vi "configuration UI.vi"() -> ()   [LabVIEW 2013, in "Tag Bus Web Interface editor node.lvclass"]
uses:
  Tag Bus Web Interface editor node.lvclass
  <vilib>/CEF_TreeControl/Node/NodeRef.ctl
  <vilib>/CEF_TreeControl/Node/NISE_CEF_Node.lvclass
  <vilib>/NI/AMC/Message Queue.ctl
  <vilib>/NI/AMC/Message.ctl
  <vilib>/NI/Tools/Keyed Array/KeyedArray.ctl
  <vilib>/CEF_TreeControl/Node/UserEventRef.ctl
  <vilib>/CEF_TreeControl/Controls/EventCluster.ctl
  <vilib>/NI/TBM Modules/TBWI/configuration/Tag Bus Web Interface configuration.lvclass
  <vilib>/NI/Module Execution Interface/Engine Configuration/engine configuration.lvclass
  <vilib>/NI/Tag Bus Data Framework/Configuration Editor/Classes/Engine Parent/Engine Parent Editor Node.lvclass
  <vilib>/NI/Tag Bus/tag/tag descriptor.lvclass
  <vilib>/NI/Tag Bus/tag/Data Type.ctl
  <vilib>/NI/Tag Bus/tag/tag descriptor.lvclass/tag descriptor.ctl
  <vilib>/NI/Tag Bus Module Framework/root configuration/TBM configuration.lvclass/TBM configuration.ctl
  <vilib>/NI/Tag Bus Module Framework/channel/channel classification.ctl
  <vilib>/NI/Tag Bus/tag/write tag name.vi
  <vilib>/NI/Tag Bus/tag/write data type.vi
  <vilib>/NI/Tag Bus Module Framework/root configuration/Read instance name.vi
  <vilib>/NI/Tag Bus/tag/read tag name.vi
  <vilib>/NI/Tag Bus Data Framework/Configuration Editor/Classes/Engine Parent/read engine configuration.vi
  <vilib>/NI/Tag Bus Data Framework/Configuration Editor/Classes/Module editor node/Read Module Configuration.vi
  <vilib>/NI/Tag Bus Module Framework/root configuration/create GUID.vi
  <vilib>/NI/Tag Bus Module Framework/root configuration/TBM configuration.lvclass
  <vilib>/NI/Tag Bus Module Framework/module configuration/TBM module configuration.lvclass
  <vilib>/NI/Tag Bus Data Framework/Configuration Editor/Classes/Module editor node/module editor node.lvclass
  <vilib>/CEF_TreeControl/NISE_CEF_TreeControl.lvlib
  <vilib>/NI/Tag Bus Module Framework/channel/TBM channel.lvclass
  <vilib>/NI/Tools/Keyed Array/Tools_KeyedArray.lvlib
  <vilib>/NI/AMC/AMC.lvlib
panel:
  in  "Tab Control":enum32{"Web Configuration"}(tab)
  in  "remove to":bool
  in  "add to":bool
  in  "remove from":bool
  in  "add from":bool
  in  "toTBWlist":i32(listbox)
  in  "fromTBWlist":i32(listbox)
  in  "avail tags":i32(listbox)=-1
  in  "Direction":enum32{"From TBWI", "To TBWI"}(radio)
  in  "user event":T1
  in  "main queue":T2
  in  "node ref":T3
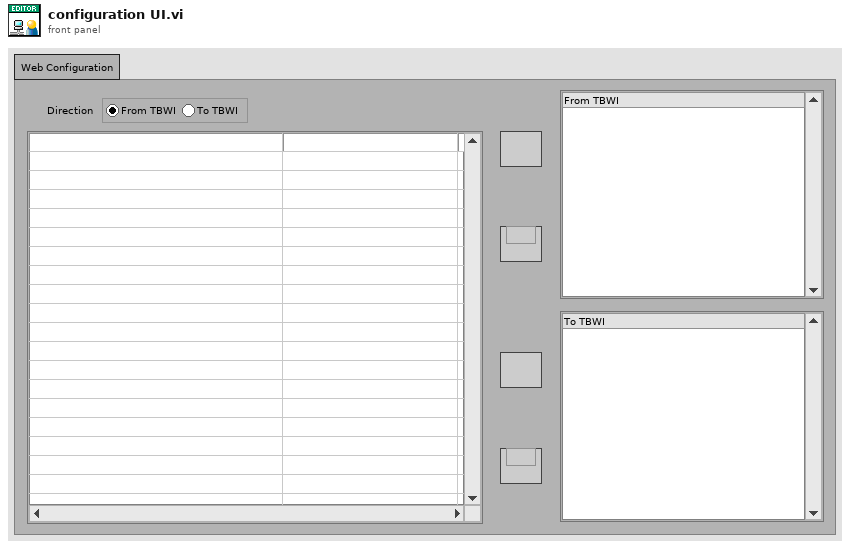
[diagram p1: front panel]
types:
  T1 = typedef "NISE_CEF_Node.lvclass/UserEventRef.ctl" = refnum<user-event>
  T2 = typedef "AMC.lvlib/Message Queue.ctl" = refnum<queue>
  T3 = typedef "NISE_CEF_Node.lvclass/NodeRef.ctl" = refnum<data-value>
  T4 = typedef "tag bus.lvlib/tag descriptor.lvclass/Data Type.ctl" = enum16{"Double", "Single", "I64", "I32", "I16", "I8", "U64", "U32", "U16", "U8", "Boolean", "String", "Array of Double", "Array of Single", "Array of I64", "Array of I32", "Array of I16", "Array of I8", "Array of U64", "Array of U32", "Array of U16", "Array of U8", "Array of Boolean", "Array of String"}
  T5 = typedef "NISE_CEF_TreeControl.lvlib/EventCluster.ctl" = cluster{"command":string, "data":string}
  T6 = enum8{"Enabled", "Disabled", "Disabled and Grayed Out"}
  T7 = typedef "TBM channel.lvclass/channel classification.ctl" = enum16{"input data", "output data", "processing parameter", "processing result"}
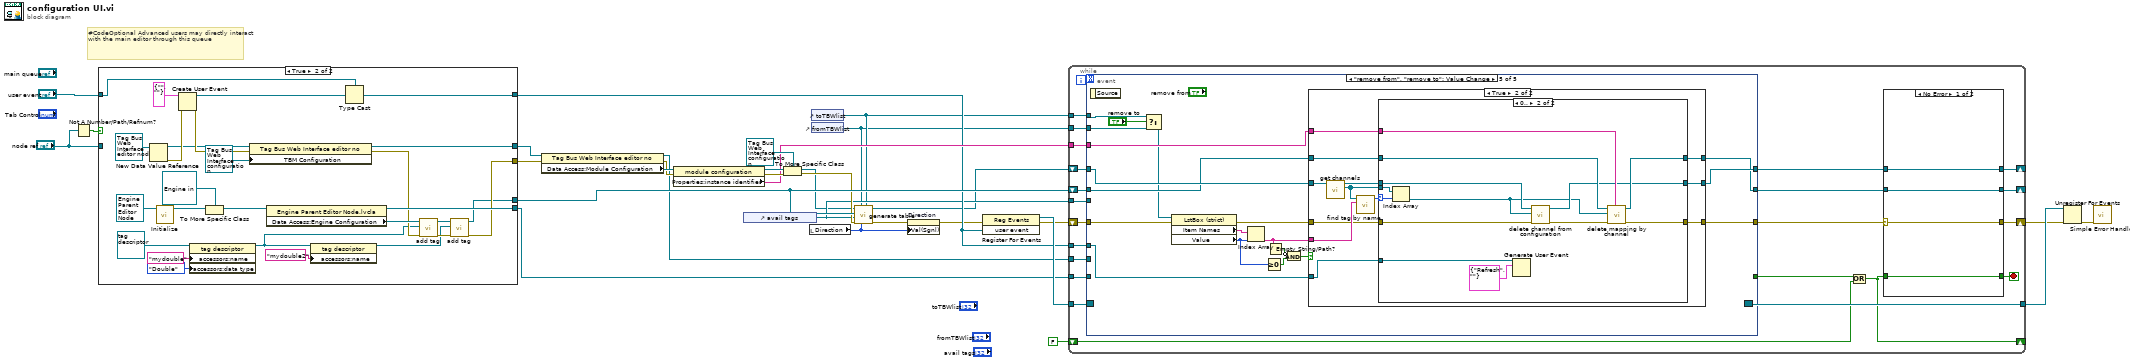
[diagram p0: block diagram]
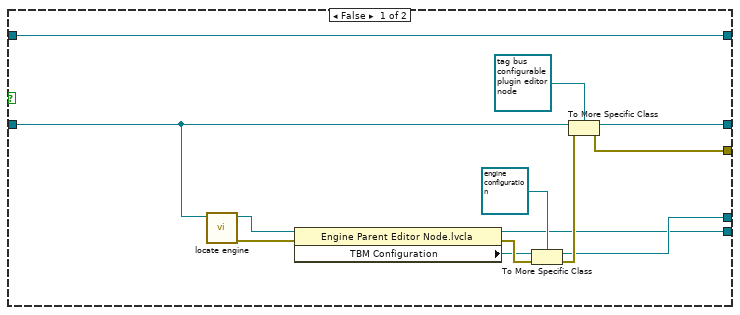
[diagram p2: hidden frame]
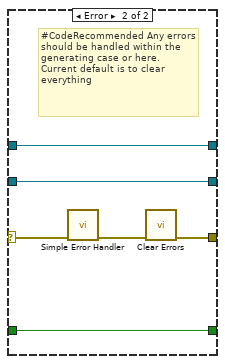
[diagram p3: hidden frame]
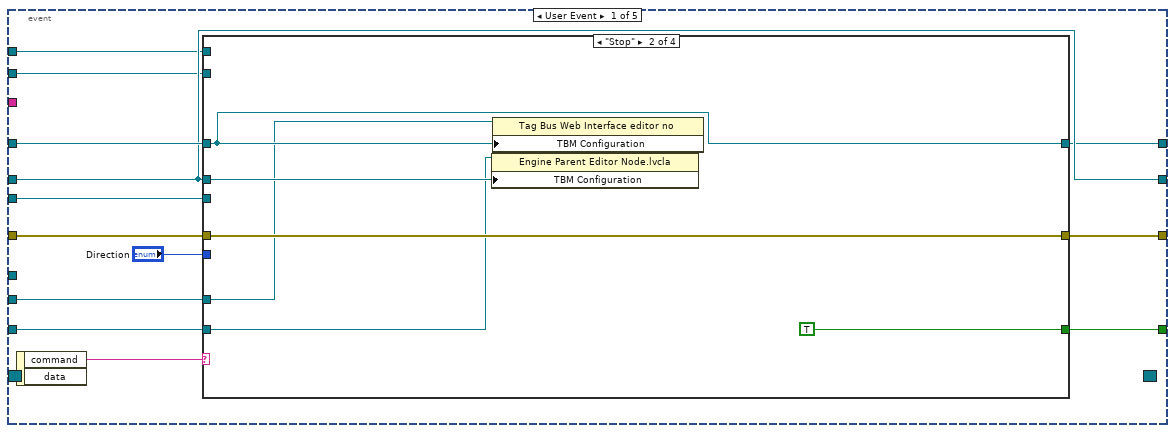
[diagram p4: hidden frame]
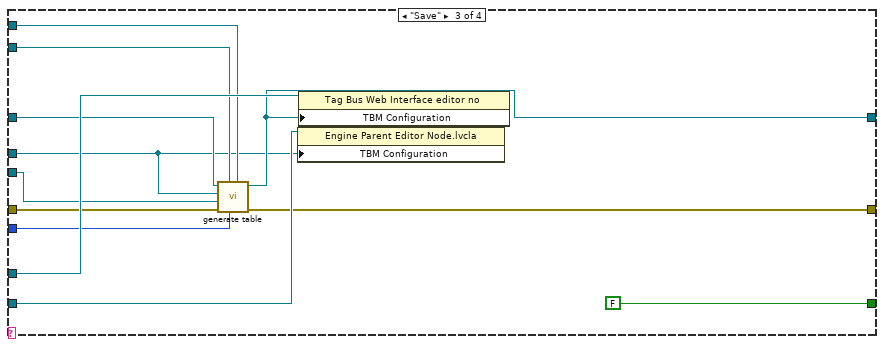
[diagram p6: hidden frame]
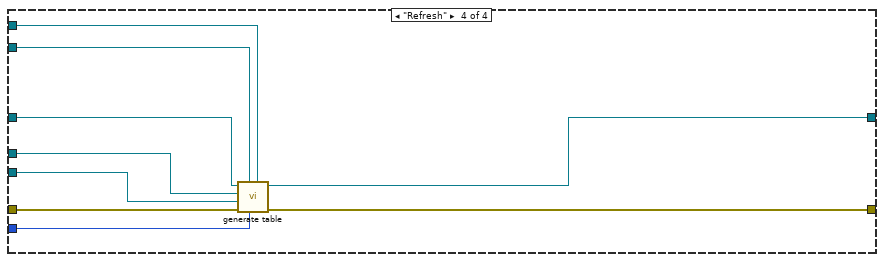
[diagram p7: hidden frame]
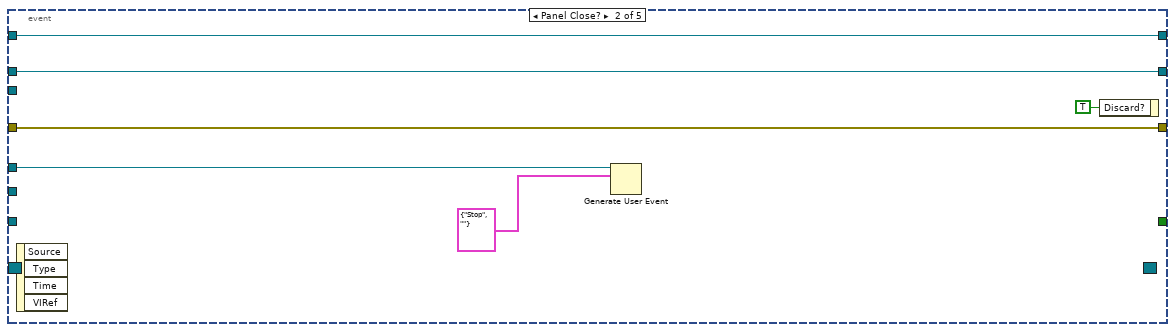
[diagram p8: hidden frame]
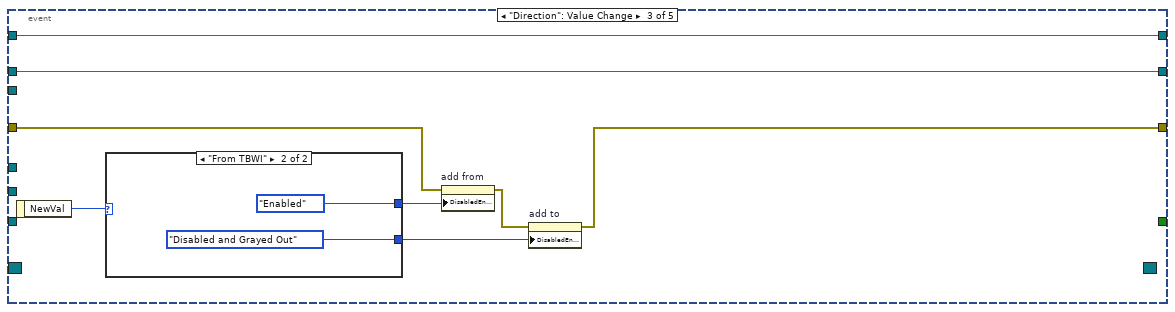
[diagram p9: hidden frame]
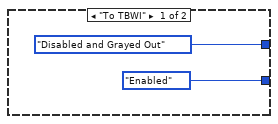
[diagram p10: hidden frame]
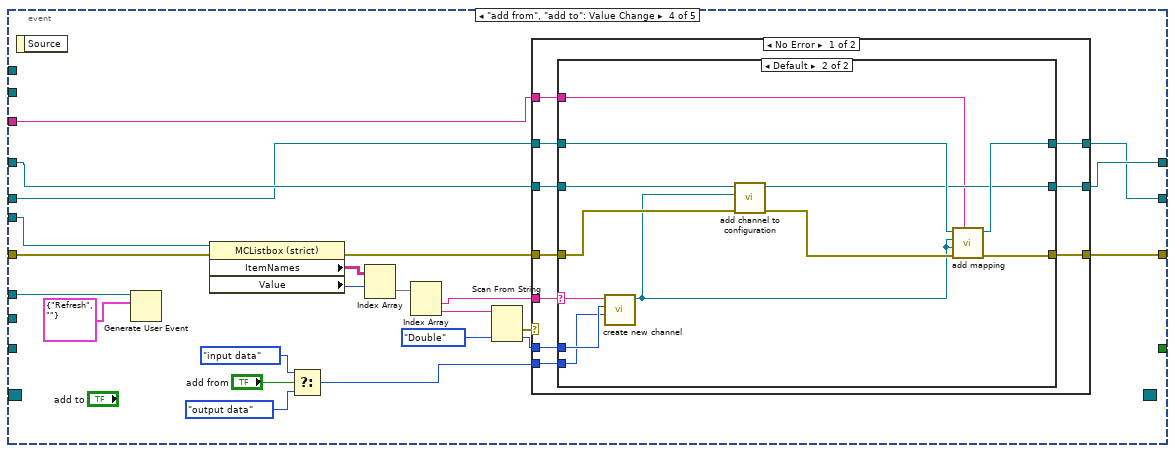
[diagram p11: hidden frame]
diagram:
  # "#CodeOptional Advanced users may directly interact with the main editor through this queue"
  n1 = Not A Number/Path/Refnum?(number/path/refnum="node ref") -> (NaN/Path/Refnum?=w21:bool)
  n2 = case shown="True" w21 {
    tunnel: "user event" -> [w43 w44]
    tunnel: [w43 w45] -> w9
    tunnel: "node ref" -> [w41 _]
    tunnel: [w40 w64] -> w14
    tunnel: [w39 w49] -> w19
    tunnel: [w32 w48] -> w16
    tunnel: [w31 w58] -> w10
    frame False {
      n3 = call <vilib>:"locate engine.vi"("component"=w41) -> ("error out"=w36:errorcluster, "engine"=w38:refnum<data-value>)  [unwired: 9 in]
      n4 = property class="Engine Parent Editor Node.lvcla"(reference=w38, error in=w36) -> (reference out=w31:refnum<data-value>, error out=w35:errorcluster, "TBM Configuration"=w34:refnum<class "TBM configuration.lvclass">)
      n5 = To More Specific Class(target class=refnum<class "engine configuration.lvclass"> refnum ("engine configuration.lvclass"), reference=w34, error in=w35) -> (specific class reference=w32:refnum<class "engine configuration.lvclass">, error out=w33:errorcluster)
      n6 = To More Specific Class(target class=refnum<data-value> refnum ("data value reference"), reference=w41, error in=w33) -> (specific class reference=w40:refnum<data-value>, error out=w39:errorcluster)
    }
    frame True {
      n7 = New Data Value Reference(data value=refnum<class "Tag Bus Web Interface editor node.lvclass"> refnum ("tag bus configurable plugin editor node")) -> (data value reference=w63:refnum<data-value>, error out=w66:errorcluster)  [unwired: 1 in]
      n8 = call-dynamic "Initialize.vi"("Engine in"=refnum<class "Engine Parent Editor Node.lvclass"> refnum) -> ("data value reference"=w62:T3)  [unwired: 8 in, 2 out]
      n9 = Create User Event(user event datatype=T5 {"command"="", "data"=""} ("event data"), error in=w66) -> (user event=w69:refnum<user-event>, error out=w65:errorcluster)
      n10 = property class="tag descriptor"(reference=refnum<class "tag descriptor.lvclass"> refnum ("tag descriptor"), "accessors:name"="mydouble" ("name"), "accessors:data type"=Data_Type."Double" ("data type")) -> (reference out=w46:refnum<class "tag descriptor.lvclass">)  [unwired: 1 in, 1 out]
      n11 = To More Specific Class(target class=refnum<data-value> refnum ("data value reference"), reference=w62) -> (specific class reference=w61:refnum<data-value>)  [unwired: 1 in, 1 out]
      n12 = property class="Tag Bus Web Interface editor no"(reference=w63, error in=w65, "TBM Configuration"=refnum<class "Tag Bus Web Interface configuration.lvclass"> refnum ("tag bus configurable plugin module configuration")) -> (reference out=w64:refnum<data-value>, error out=w53:errorcluster)
      n13 = property class="Engine Parent Editor Node.lvcla"(reference=w61) -> (reference out=w58:refnum<data-value>, "Data Access:Engine Configuration"=w57:refnum<class "engine configuration.lvclass">)  [unwired: 1 in, 1 out]
      n14 = property class="tag descriptor"(reference=w46, "accessors:name"="mydouble2" ("name")) -> (reference out=w47:refnum<class "tag descriptor.lvclass">)  [unwired: 1 in, 1 out]
      n15 = Type Cast(type=w44, x=w69) -> (*(type *) &x=w45:T1)
      n16 = call <vilib>:"add tag.vi"("error in"=w53, "tag descriptor"=w46, "engine configuration in"=w57) -> ("error out"=w51:errorcluster, "engine configuration out"=w50:refnum<class "engine configuration.lvclass">)  [unwired: 7 in]
      n17 = call <vilib>:"add tag.vi"("error in"=w51, "tag descriptor"=w47, "engine configuration in"=w50) -> ("error out"=w49:errorcluster, "engine configuration out"=w48:refnum<class "engine configuration.lvclass">)  [unwired: 7 in]
    }
  }
  n18 = property class="Tag Bus Web Interface editor no"(reference=w14, error in=w19) -> (reference out=w11:refnum<data-value>, error out=w24:errorcluster, "Data Access:Module Configuration"=w25:refnum<class "TBM module configuration.lvclass">)
  n19 = property class="module configuration"(reference=w25, error in=w24) -> (reference out=w22:refnum<class "TBM module configuration.lvclass">, error out=w23:errorcluster, "Properties:instance identifier"=w18:string)
  n20 = control-ref of="avail tags"() -> (w8:refnum<vi>)
  n21 = To More Specific Class(target class=refnum<class "Tag Bus Web Interface configuration.lvclass"> refnum ("tag bus configurable plugin module configuration"), reference=w22, error in=w23) -> (specific class reference=w7:refnum<class "Tag Bus Web Interface configuration.lvclass">, error out=w15:errorcluster)
  n22 = local read "Direction"() -> (w1:enum32{"From TBWI", "To TBWI"})
  n23 = control-ref of="toTBWlist"() -> (w5:refnum<vi>)
  n24 = control-ref of="fromTBWlist"() -> (w4:refnum<vi>)
  n25 = call "generate table.vi"("to tbwi"=w5, "Direction"=w1, "from tbwi"=w4, "error in"=w15, "tags"=w8, "engine configuration in"=w16, "Tag Bus Web Interface configuration in"=w7) -> ("error out"=w3:errorcluster, "TBWI Cfg out"=w6:refnum<class "Tag Bus Web Interface configuration.lvclass">)  [unwired: 3 in]
  n26 = property on="Direction" class="RadioBtnsControl (strict)"(error in=w3, "Val(Sgnl)"=w1) -> (error out=w2:errorcluster)  [unwired: 1 in, 1 out]
  n27 = register-events(error in=w2, w9) -> (reference out=w30:refnum<event-registration>, error out=w13:errorcluster)  [unwired: 1 in]
  n28 = while {
    tunnel: w30 -> [w92]
    tunnel: [w91] -> w29
    shift-right: [w85] -> w28
    shift-left: w13 -> [w90]
    shift-right: [w87] -> _
    shift-left: FALSE -> [w86]
    shift-right: [w81] -> _
    shift-left: w6 -> [w84]
    shift-right: [w82] -> _
    shift-left: w16 -> [w83]
    tunnel: w18 -> [w80]
    tunnel: w11 -> [w76]
    tunnel: w10 -> [w75]
    tunnel: w8 -> [w74]
    tunnel: w9 -> [w73]
    tunnel: w5 -> [w72]
    tunnel: w4 -> [w71]
    stop <- w89 stop-if-true
    n29 = event shown="[4] \"remove from\", \"remove to\": Value Change" {
      selector: w92 -> [_ _ _ _ _]
      dyn-events: [_ _ _ _ _] -> w91
      timeout: _ -> [_ _ _ _ _]
      tunnel: [w115 _ _ _ _] -> w88
      tunnel: [w113 w150 w151 w164 w222] -> w77
      tunnel: w90 -> [w112 w150 w152 w171 w215]
      tunnel: w84 -> [w111 w145 w157 w169 w219]
      tunnel: w83 -> [w110 w146 w158 w168 w218]
      tunnel: [w110 w146 w158 w165 w220] -> w79
      tunnel: [w106 w145 w157 w166 w221] -> w78
      tunnel: w80 -> [_ _ _ w167 w217]
      tunnel: w76 -> [w109 _ _ _ _]
      tunnel: w75 -> [w108 _ _ _ _]
      tunnel: w74 -> [w107 _ _ w170 _]
      tunnel: w73 -> [_ w148 _ w185 w214]
      tunnel: w72 -> [w104 _ _ _ w232]
      tunnel: w71 -> [w105 _ _ _ w230]
      event User Event {
        n30 = event-data() -> ("command"=w114:string)  [unwired: 1 in, 1 out]
        n31 = case shown="\"Stop\"" w114 {
          tunnel: [_ TRUE FALSE _] -> w115
          tunnel: [w117 w122 w124 w141] -> w113
          tunnel: w112 -> [w117 w122 w132 w144]
          tunnel: w111 -> [w116 w121 w131 w143]
          tunnel: w110 -> [_ w120 w127 w142]
          tunnel: w109 -> [_ w119 w134 _]
          tunnel: w108 -> [_ w118 w133 _]
          tunnel: w107 -> [_ _ w126 w136]
          tunnel: [w116 w121 w130 w140] -> w106
          tunnel: w105 -> [_ _ w128 w139]
          tunnel: w104 -> [_ _ w129 w138]
          tunnel: "Direction" -> [_ _ w125 w137]
          frame Default {
          }
          frame "Stop" {
            n32 = property class="Engine Parent Editor Node.lvcla"(reference=w118, "TBM Configuration"=w120) -> ()  [unwired: 1 in, 2 out]
            n33 = property class="Tag Bus Web Interface editor no"(reference=w119, "TBM Configuration"=w121) -> ()  [unwired: 1 in, 2 out]
          }
          frame "Save" {
            n34 = call "generate table.vi"("to tbwi"=w129, "Direction"=w125, "from tbwi"=w128, "error in"=w132, "tags"=w126, "engine configuration in"=w127, "Tag Bus Web Interface configuration in"=w131) -> ("error out"=w124:errorcluster, "TBWI Cfg out"=w130:refnum<class "Tag Bus Web Interface configuration.lvclass">)  [unwired: 3 in]
            n35 = property class="Engine Parent Editor Node.lvcla"(reference=w133, "TBM Configuration"=w127) -> ()  [unwired: 1 in, 2 out]
            n36 = property class="Tag Bus Web Interface editor no"(reference=w134, "TBM Configuration"=w130) -> ()  [unwired: 1 in, 2 out]
          }
          frame "Refresh" {
            n37 = call "generate table.vi"("to tbwi"=w138, "Direction"=w137, "from tbwi"=w139, "error in"=w144, "tags"=w136, "engine configuration in"=w142, "Tag Bus Web Interface configuration in"=w143) -> ("error out"=w141:errorcluster, "TBWI Cfg out"=w140:refnum<class "Tag Bus Web Interface configuration.lvclass">)  [unwired: 3 in]
          }
        }
      }
      event Panel Close? {
        n38 = event-data() -> ()  [unwired: 1 in, 4 out]
        n39 = Generate User Event(user event=w148, event data cluster=T5 {"command"="Stop", "data"=""} ("event data")) -> ()  [unwired: 2 in, 2 out]
        n40 = event-data("Discard?"=TRUE) -> ()  [unwired: 1 in, 1 out]
      }
      event "Direction": Value Change {
        n41 = event-data() -> ("NewVal"=w156:enum32{"From TBWI", "To TBWI"})  [unwired: 1 in]
        n42 = case shown="\"From TBWI\"" w156 {
          tunnel: [T6."Disabled and Grayed Out" ("Disabled") T6."Enabled" ("Disabled")] -> w155
          tunnel: [T6."Enabled" ("Disabled") T6."Disabled and Grayed Out" ("Disabled")] -> w154
          frame "To TBWI" {
          }
          frame "From TBWI" {
          }
        }
        n43 = property on="add from" class="Bool"(error in=w152, "DisabledEnum"=w155) -> (error out=w153:errorcluster)  [unwired: 1 in, 1 out]
        n44 = property on="add to" class="Bool"(error in=w153, "DisabledEnum"=w154) -> (error out=w151:errorcluster)  [unwired: 1 in, 1 out]
      }
      event "add from", "add to": Value Change {
        n45 = event-data() -> ()  [unwired: 1 in, 1 out]
        n46 = Generate User Event(user event=w185, event data cluster=T5 {"command"="Refresh", "data"=""} ("event data")) -> ()  [unwired: 2 in, 2 out]
        n47 = property class="MCListbox (strict)"(reference=w170, error in=w171) -> (error out=w172:errorcluster, "ItemNames"=w173:string[][], "Value"=w174:i32)  [unwired: 1 out]
        n48 = Select(t=channel_classification."input data" ("channel classification"), s="add from", f=channel_classification."output data" ("channel classification")) -> (s? t:f=w163:T7)
        n49 = Index Array(array=w173, index (row)=w174) -> (element=w177:string[])  [unwired: 1 in]
        n50 = Index Array(array=w177) -> (element #1=w178:string, element #2=w175:string)  [unwired: 2 in]
        n51 = Scan From String(input string=w175, default 1=Data_Type."Double" ("data type")) -> (error out=w179:errorcluster, output 1=w180:T4)  [unwired: 3 in, 2 out]
        n52 = case shown="No Error" w179 {
          tunnel: [w195 w211] -> w164
          tunnel: w167 -> [w194 _]
          tunnel: [w193 w213] -> w165
          tunnel: [w192 w212] -> w166
          tunnel: w169 -> [w191 w212]
          tunnel: w168 -> [w190 w213]
          tunnel: w172 -> [w189 w211]
          tunnel: w178 -> [w188 _]
          tunnel: w180 -> [w187 _]
          tunnel: w163 -> [w186 _]
          frame No Error {
            n53 = case shown="Default" w188 {
              selector: w188 -> [_ w202]
              tunnel: [w198 w210] -> w195
              tunnel: w189 -> [w198 w205]
              tunnel: w190 -> [w196 w209]
              tunnel: [w197 w206] -> w192
              tunnel: w191 -> [w197 w207]
              tunnel: [w196 w208] -> w193
              tunnel: w194 -> [_ w203]
              tunnel: w187 -> [_ w201]
              tunnel: w186 -> [_ w199]
              frame "" {
              }
              frame Default {
                n54 = call <vilib>:"create new channel.vi"("channel classification"=w199, "data type"=w201, "channel name"=w202) -> ("channel"=w200:refnum<class "TBM channel.lvclass">)  [unwired: 8 in]
                n55 = call <vilib>:"add channel to configuration.vi"("error in"=w205, "TBM channel in"=w200, "Tag Bus Web Interface configuration in"=w207) -> ("error out"=w204:errorcluster, "Tag Bus Web Interface configuration out"=w206:refnum<class "Tag Bus Web Interface configuration.lvclass">)  [unwired: 7 in]
                n56 = call <vilib>:"add mapping.vi"("owner ID"=w203, "error in"=w204, "channel"=w200, "tag descriptor"=w200, "engine configuration"=w209) -> ("error out"=w210:errorcluster, "engine configuration out"=w208:refnum<class "engine configuration.lvclass">)  [unwired: 5 in]
              }
            }
          }
          frame Error {
          }
        }
      }
      event "remove from", "remove to": Value Change {
        n57 = event-data() -> ()  [unwired: 1 in, 1 out]
        n58 = Select(t=w232, s="remove to", f=w230) -> (s? t:f=w216:refnum<vi>)
        n59 = property class="LstBox (strict)"(reference=w216, error in=w215) -> (error out=w228:errorcluster, "Item Names"=w223:string[], "Value"=w224:i32)  [unwired: 1 out]
        n60 = Index Array(array=w223, index=w224) -> (element=w229:string)
        n61 = Greater Or Equal To 0?(x=w224) -> (x >= 0?=w226:bool)
        n62 = Empty String/Path?(string/path=w229) -> (empty?=w225:bool)
        n63 = Compound Arithmetic op=AND(invert w225, w226) -> (w227:bool)
        n64 = case shown="True" w227 {
          tunnel: w228 -> [w235 w240]
          tunnel: [w235 w241] -> w222
          tunnel: w219 -> [w234 w246]
          tunnel: [w234 w242] -> w221
          tunnel: [w233 w238] -> w220
          tunnel: w218 -> [w233 w239]
          tunnel: w214 -> [_ w247]
          tunnel: w229 -> [_ w245]
          tunnel: w217 -> [_ w236]
          frame False {
          }
          frame True {
            n65 = call-dynamic "get channels.vi"("Tag Bus Web Interface configuration in"=w246) -> ("channels"=w237:refnum<class "TBM channel.lvclass">[], "Tag Bus Web Interface configuration out"=w243:refnum<class "Tag Bus Web Interface configuration.lvclass">)  [unwired: 9 in]
            n66 = call <vilib>:"find tag by name.vi"("name"=w245, "tags in"=w237) -> ("index"=w244:i32)  [unwired: 9 in]
            n67 = case shown="0.." w244 {
              selector: w244 -> [_ w261]
              tunnel: w247 -> [_ w262]
              tunnel: w243 -> [w250 w259]
              tunnel: [w250 w253] -> w242
              tunnel: [w249 w252] -> w241
              tunnel: w240 -> [w249 w258]
              tunnel: w239 -> [w248 w257]
              tunnel: [w248 w254] -> w238
              tunnel: w237 -> [_ w260]
              tunnel: w236 -> [_ w255]
              frame ..-1 {
              }
              frame 0.. {
                n68 = Index Array(array=w260, index=w261) -> (element=w251:refnum<class "TBM channel.lvclass">)
                n69 = Generate User Event(user event=w262, event data cluster=T5 {"command"="Refresh", "data"=""} ("event data")) -> ()  [unwired: 2 in, 2 out]
                n70 = call <vilib>:"delete channel from configuration.vi"("error in"=w258, "TBM channel in"=w251, "Tag Bus Web Interface configuration in"=w259) -> ("error out"=w256:errorcluster, "Tag Bus Web Interface configuration out"=w253:refnum<class "Tag Bus Web Interface configuration.lvclass">)  [unwired: 7 in]
                n71 = call <vilib>:"delete mapping by channel.vi"("owner ID"=w255, "error in"=w256, "channel"=w251, "engine configuration in"=w257) -> ("error out"=w252:errorcluster, "engine configuration out"=w254:refnum<class "engine configuration.lvclass">)  [unwired: 6 in]
              }
            }
          }
        }
      }
    }
    n72 = Or(x=w88, y=w86) -> (x .or. y?=w87:bool)
    n73 = case shown="No Error" w77 {
      selector: w77 -> [w93 w101]
      tunnel: [w96 w102] -> w89
      tunnel: w87 -> [w96 w102]
      tunnel: [w93 w99] -> w85
      tunnel: w79 -> [w94 w98]
      tunnel: [w94 w98] -> w82
      tunnel: w78 -> [w95 w97]
      tunnel: [w95 w97] -> w81
      frame No Error {
      }
      frame Error {
        # "#CodeRecommended Any errors should be handled within the generating case or here. Current default is to clear everything"
        n74 = call <vilib>:"Simple Error Handler.vi"("error in (no error)"=w101) -> ("error out"=w100:errorcluster)  [unwired: 4 in, 4 out]
        n75 = call <vilib>:"Clear Errors.vi"("error in (no error)"=w100) -> ("error out"=w99:errorcluster)  [unwired: 6 in]
      }
    }
  }
  n76 = Unregister For Events(event registration refnum=w29, error in=w28) -> (error out=w12:errorcluster)
  n77 = call <vilib>:"Simple Error Handler.vi"("error in (no error)"=w12) -> ()  [unwired: 4 in, 5 out]
